vi "Test Air Leak ODBC.vi"() -> ()   [LabVIEW 2013]
uses:
  Controls/ALTS-2015 Obtain Test Data DB Driver Options.ctl
  Controls/ALTS-2015 Station Cluster.ctl
panel:
  out "data":string[][](array[string])
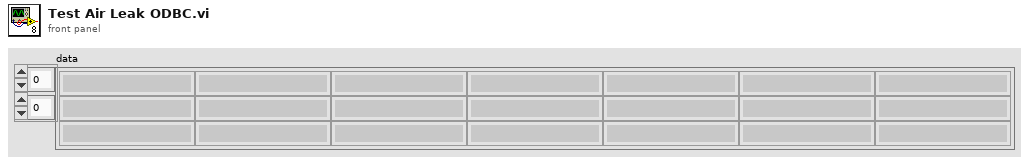
[diagram p1: front panel]
types:
  T1 = typedef "ALTS-2015 Station Cluster.ctl" = enum16{"Station 1", "Station 2", "Station 3", "Station 4"}
  T2 = typedef "ALTS-2015 Obtain Test Data DB Driver Options.ctl" = enum16{"Init", "Read Test Data Results", "Close"}
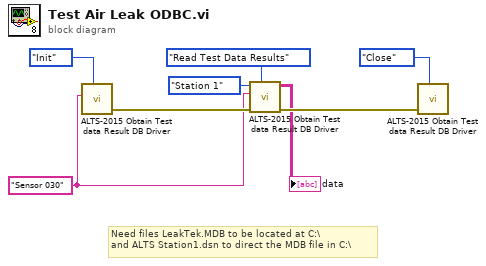
[diagram p0: block diagram]
diagram:
  w2 = "Sensor 030" ("Sensor Name")
  # "Need files LeakTek.MDB to be located at C:\\\nand ALTS Station1.dsn to direct the MDB file in C:\\"
  n1 = call "ALTS-2015 Obtain Test data Result DB Driver.vi"("Option"=ALTS-2015_Obtain_Test_Data_DB_Driver_Options."Init", "Sensor Name"=w2) -> ("error out"=w7:errorcluster)  [unwired: 8 in, 1 out]
  n2 = call "ALTS-2015 Obtain Test data Result DB Driver.vi"("Option"=ALTS-2015_Obtain_Test_Data_DB_Driver_Options."Read Test Data Results", "error in"=w7, "Sensor Name"=w2, "Station Enum"=ALTS-2015_Station_Cluster."Station 1") -> ("error out"=w8:errorcluster, "data"=→"data":string[][])  [unwired: 6 in]
  n3 = call "ALTS-2015 Obtain Test data Result DB Driver.vi"("Option"=ALTS-2015_Obtain_Test_Data_DB_Driver_Options."Close", "error in"=w8) -> ()  [unwired: 8 in, 2 out]
